vi "Ejemplo3_fuentes.vi"() -> ()   [LabVIEW 2020]
panel:
  in  "String 6":string
  out "Boolean 6":bool
  in  "Numeric 6":dbl
  out "Cluster 4":T1 {"Thermometer" scale=0.0..100.0}
  out "Array 4":bool[](array[boolean])
  in  "String 5":string
  out "Boolean 5":bool
  in  "Numeric 5":dbl
  in  "Boolean 4":bool
  in  "String 4":string
  in  "Numeric 4":dbl
  out "Array 3":bool[](array[boolean])
  out "Cluster 3":T1 {"Thermometer" scale=0.0..100.0}
  in  "String 3":string
  out "Boolean 3":bool
  in  "Numeric 3":dbl
  in  "Cluster 2":T2 {"Tank" scale=0.0..10.0}
  out "Array 2":bool[](array[boolean])
  in  "String 2":string
  out "Boolean 2":bool
  in  "Numeric 2":dbl
  out "Cluster":T1 {"Thermometer" scale=0.0..100.0}
  out "Array":bool[](array[boolean])
  in  "String":string
  out "Boolean":bool
  in  "Numeric":dbl
  # "Fuentes"
  # "Nxg Style"
  # "Silver"
  # "Modern"
  # "Classic"
  # "Express"
  # "System"
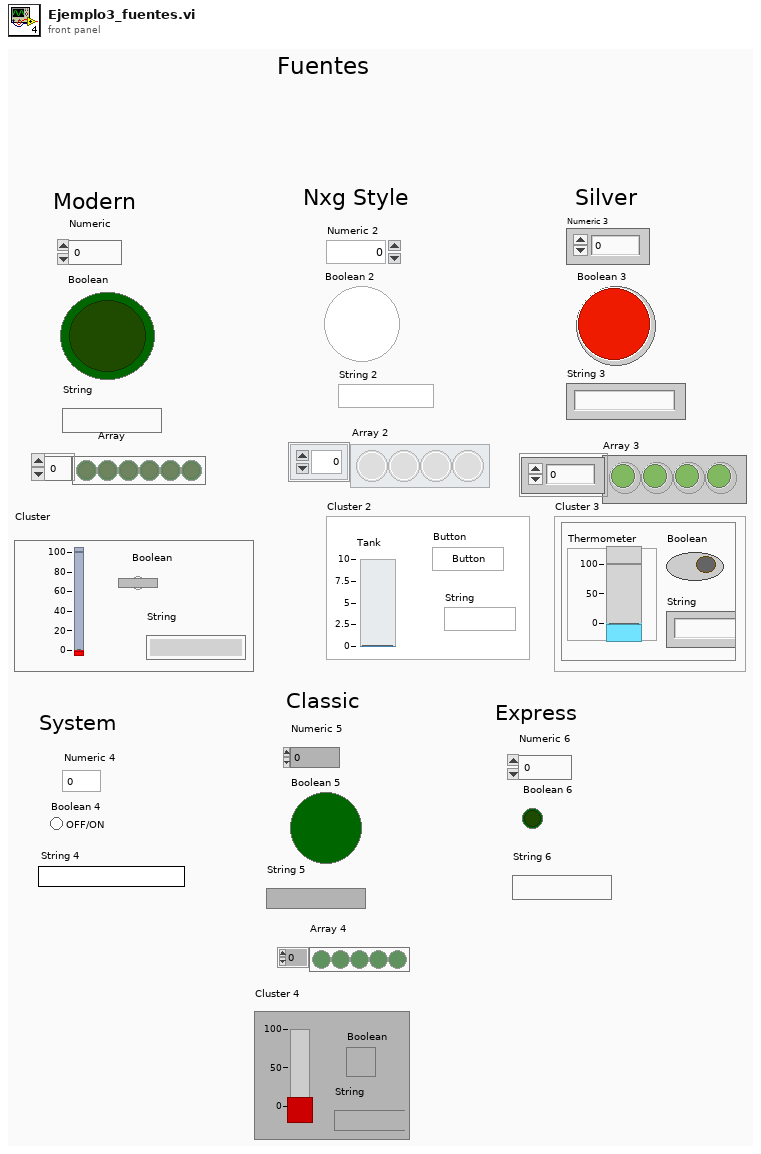
[diagram p1: front panel]
types:
  T1 = cluster{"Thermometer":dbl, "Boolean":bool, "String":string}
  T2 = cluster{"Tank":dbl, "Button":bool, "String":string}
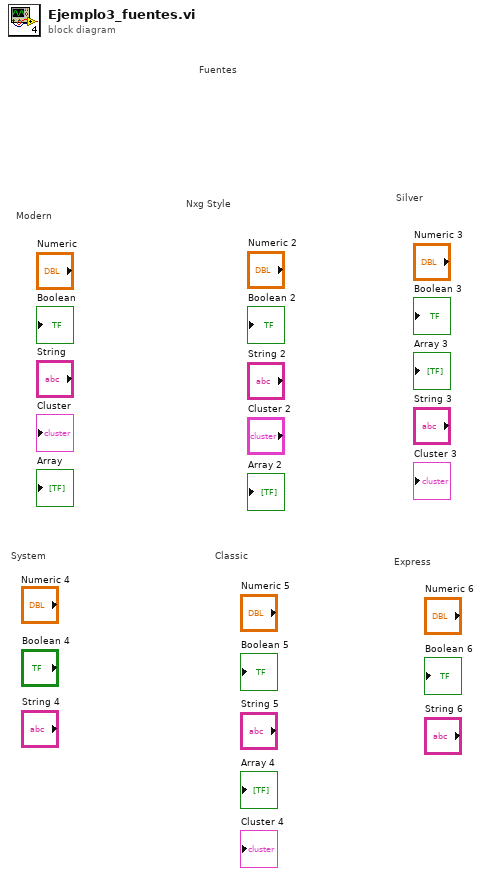
[diagram p0: block diagram]
diagram:
  # "Fuentes"
  # "Express"
  # "Classic"
  # "System"
  # "Silver"
  # "Nxg Style"
  # "Modern"
